vi "CountShantenWithoutEye.vi"(1 "HandCount":u16[](array[numeric])) -> (0 "shanten":u16)   [LabVIEW 2025]
panel:
  in  "VI Refnum":refnum<vi>
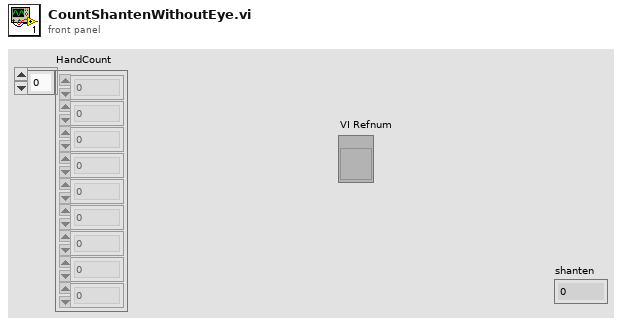
[diagram p1: front panel]
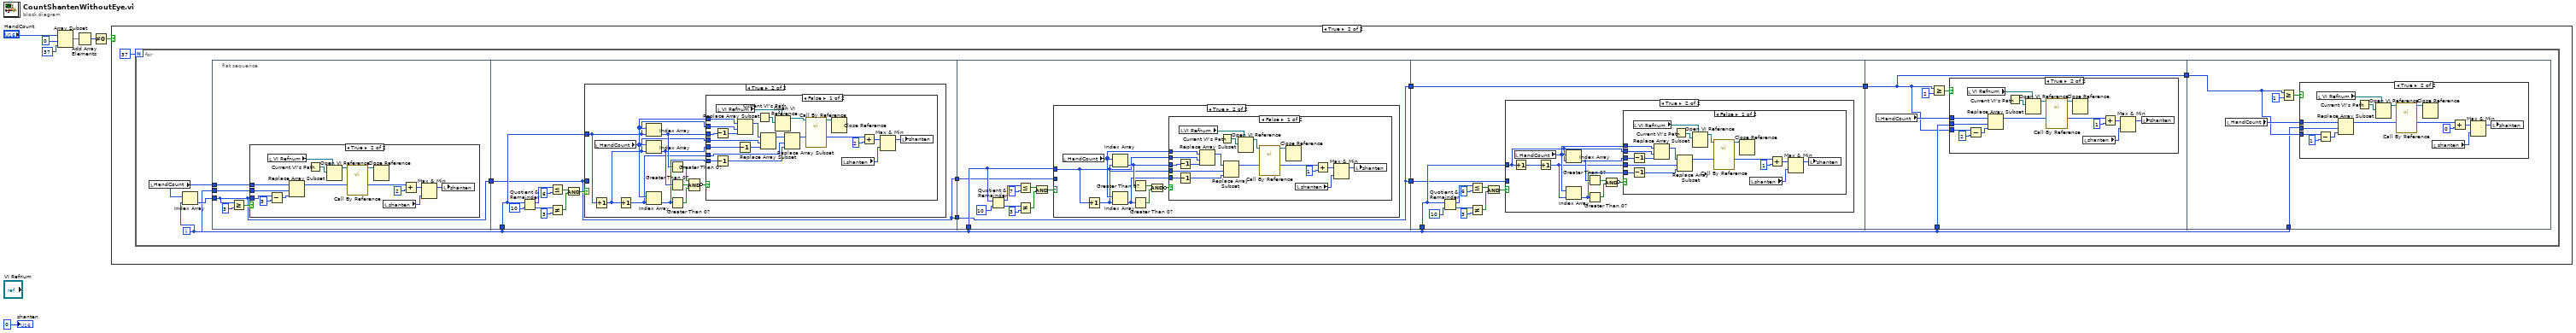
[diagram p0: block diagram]
diagram:
  n1 = Array Subset(array="HandCount", index=0, length=37) -> (w4:u16[])
  n2 = Add Array Elements(numeric array=w4) -> (sum=w2:u16)
  n3 = Not Equal To 0?(x=w2) -> (x != 0?=w3:bool)
  n4 = case shown="True" w3 {
    frame False {
    }
    frame True {
      n5 = for {
        N: 37 -> [_]
        i -> [w9]
        n6 = local read "HandCount"() -> (w16:u16[])
        n7 = Index Array(array=w16, index=w9) -> (element=w18:u16)
        n8 = flat-sequence {
          tunnel: w18 -> [w19]
          tunnel: [w19] -> w17
          tunnel: w16 -> [w21]
          tunnel: w9 -> [w20]
          tunnel: w17 -> [w39]
          tunnel: w9 -> [w41]
          tunnel: [w39] -> w15
          tunnel: [w39] -> w13
          tunnel: w9 -> [w84]
          tunnel: w15 -> [w83]
          tunnel: [w82] -> w14
          tunnel: w13 -> [w82]
          tunnel: [w82] -> w11
          tunnel: w9 -> [w121]
          tunnel: w14 -> [w120]
          tunnel: [w119] -> w12
          tunnel: w11 -> [w119]
          tunnel: w12 -> [w157]
          tunnel: w9 -> [w158]
          tunnel: [w157] -> w10
          tunnel: w10 -> [w178]
          tunnel: w9 -> [w177]
          frame #0 {
            n9 = Greater Or Equal?(x=w19, y=3) -> (x >= y?=w23:bool)
            n10 = case shown="True" w23 {
              tunnel: w21 -> [_ w38]
              tunnel: w20 -> [_ w37]
              tunnel: w19 -> [_ w34]
              frame False {
              }
              frame True {
                n11 = local read "VI Refnum"() -> (w32:refnum<vi>)
                n12 = Subtract(x=w34, y=3) -> (x-y=w35:i32)
                n13 = Replace Array Subset(array=w38, new element=w35, index=w37) -> (w30:u16[])
                n14 = Current VI's Path() -> (path=w33:path)
                n15 = Open VI Reference(type specifier VI Refnum (for type only)=w32, vi path=w33) -> (vi reference=w31:refnum<vi>)  [unwired: 4 in, 1 out]
                n16 = call-by-ref "?"(reference=w31, "HandCount"=w30) -> (reference out=w29:refnum<vi>, "Numeric"=w27:u16)  [unwired: 1 in, 1 out]
                n17 = Close Reference(reference=w29) -> ()  [unwired: 1 in, 1 out]
                n18 = local read "shanten"() -> (w28:u16)
                n19 = Add(x=w27, y=2) -> (x+y=w25:i32)
                n20 = Max & Min(x=w25, y=w28) -> (max(x,y)=w24:i32)  [unwired: 1 out]
                n21 = local write "shanten"(w24) -> ()
              }
            }
          }
          frame #1 {
            n22 = Quotient & Remainder(x=w41, y=10) -> (x-y*floor(x/y)=w47:i32, floor(x/y)=w45:i32)
            n23 = Less Or Equal?(x=w47, y=6) -> (x <= y?=w43:bool)
            n24 = Not Equal?(x=w45, y=3) -> (x != y?=w42:bool)
            n25 = And(x=w43, y=w42) -> (x .and. y?=w40:bool)
            n26 = case shown="True" w40 {
              tunnel: w39 -> [_ _]
              tunnel: w41 -> [_ w49]
              frame False {
              }
              frame True {
                n27 = Increment(x=w49) -> (x+1=w53:i32)
                n28 = local read "HandCount"() -> (w56:u16[])
                n29 = Increment(x=w53) -> (x+1=w51:i32)
                n30 = Index Array(array=w56, index=w49) -> (element=w55:u16)
                n31 = Index Array(array=w56, index=w53) -> (element=w54:u16)
                n32 = Index Array(array=w56, index=w51) -> (element=w52:u16)
                n33 = Greater Than 0?(x=w55) -> (x > 0?=w59:bool)
                n34 = Greater Than 0?(x=w54) -> (x > 0?=w58:bool)
                n35 = Greater Than 0?(x=w52) -> (x > 0?=w57:bool)
                n36 = Compound Arithmetic op=AND(w59, w58, w57) -> (invert w50:bool)
                n37 = case shown="False" w50 {
                  tunnel: w56 -> [w79 _]
                  tunnel: w55 -> [w75 _]
                  tunnel: w54 -> [w74 _]
                  tunnel: w53 -> [w73 _]
                  tunnel: w52 -> [w72 _]
                  tunnel: w51 -> [w71 _]
                  tunnel: w49 -> [w65 _]
                  frame False {
                    n38 = Decrement(x=w75) -> (x-1=w78:u16)
                    n39 = Decrement(x=w72) -> (x-1=w76:u16)
                    n40 = local read "VI Refnum"() -> (w70:refnum<vi>)
                    n41 = Replace Array Subset(array=w79, new element=w78, index=w65) -> (w81:u16[])
                    n42 = Decrement(x=w74) -> (x-1=w77:u16)
                    n43 = Current VI's Path() -> (path=w67:path)
                    n44 = Replace Array Subset(array=w81, new element=w77, index=w73) -> (w80:u16[])
                    n45 = Open VI Reference(type specifier VI Refnum (for type only)=w70, vi path=w67) -> (vi reference=w69:refnum<vi>)  [unwired: 4 in, 1 out]
                    n46 = Replace Array Subset(array=w80, new element=w76, index=w71) -> (w66:u16[])
                    n47 = call-by-ref "?"(reference=w69, "HandCount"=w66) -> (reference out=w68:refnum<vi>, "Numeric"=w60:u16)  [unwired: 1 in, 1 out]
                    n48 = Close Reference(reference=w68) -> ()  [unwired: 1 in, 1 out]
                    n49 = local read "shanten"() -> (w64:u16)
                    n50 = Add(x=w60, y=2) -> (x+y=w63:i32)
                    n51 = Max & Min(x=w63, y=w64) -> (max(x,y)=w62:i32)  [unwired: 1 out]
                    n52 = local write "shanten"(w62) -> ()
                  }
                  frame True {
                  }
                }
              }
            }
          }
          frame #2 {
            n53 = Quotient & Remainder(x=w84, y=10) -> (x-y*floor(x/y)=w86:i32, floor(x/y)=w88:i32)
            n54 = Less Or Equal?(x=w86, y=7) -> (x <= y?=w90:bool)
            n55 = Not Equal?(x=w88, y=3) -> (x != y?=w91:bool)
            n56 = And(x=w90, y=w91) -> (x .and. y?=w92:bool)
            n57 = case shown="True" w92 {
              tunnel: w83 -> [_ _]
              tunnel: w84 -> [_ w93]
              frame False {
              }
              frame True {
                n58 = local read "HandCount"() -> (w98:u16[])
                n59 = Increment(x=w93) -> (x+1=w95:i32)
                n60 = Index Array(array=w98, index=w93) -> (element=w97:u16)
                n61 = Index Array(array=w98, index=w95) -> (element=w96:u16)
                n62 = Greater Than 0?(x=w97) -> (x > 0?=w100:bool)
                n63 = Greater Than 0?(x=w96) -> (x > 0?=w99:bool)
                n64 = Compound Arithmetic op=AND(w100, w99) -> (invert w94:bool)
                n65 = case shown="False" w94 {
                  tunnel: w98 -> [w117 _]
                  tunnel: w97 -> [w114 _]
                  tunnel: w96 -> [w113 _]
                  tunnel: w95 -> [w112 _]
                  tunnel: w93 -> [w107 _]
                  frame False {
                    n66 = Decrement(x=w114) -> (x-1=w116:u16)
                    n67 = Decrement(x=w113) -> (x-1=w115:u16)
                    n68 = local read "VI Refnum"() -> (w111:refnum<vi>)
                    n69 = Replace Array Subset(array=w117, new element=w116, index=w107) -> (w118:u16[])
                    n70 = Current VI's Path() -> (path=w108:path)
                    n71 = Replace Array Subset(array=w118, new element=w115, index=w112) -> (w101:u16[])
                    n72 = Open VI Reference(type specifier VI Refnum (for type only)=w111, vi path=w108) -> (vi reference=w110:refnum<vi>)  [unwired: 4 in, 1 out]
                    n73 = call-by-ref "?"(reference=w110, "HandCount"=w101) -> (reference out=w109:refnum<vi>, "Numeric"=w102:u16)  [unwired: 1 in, 1 out]
                    n74 = Close Reference(reference=w109) -> ()  [unwired: 1 in, 1 out]
                    n75 = local read "shanten"() -> (w106:u16)
                    n76 = Add(x=w102, y=1) -> (x+y=w105:i32)
                    n77 = Max & Min(x=w105, y=w106) -> (max(x,y)=w104:i32)  [unwired: 1 out]
                    n78 = local write "shanten"(w104) -> ()
                  }
                  frame True {
                  }
                }
              }
            }
          }
          frame #3 {
            n79 = Quotient & Remainder(x=w121, y=10) -> (x-y*floor(x/y)=w128:i32, floor(x/y)=w126:i32)
            n80 = Less Or Equal?(x=w128, y=6) -> (x <= y?=w124:bool)
            n81 = Not Equal?(x=w126, y=3) -> (x != y?=w123:bool)
            n82 = And(x=w124, y=w123) -> (x .and. y?=w122:bool)
            n83 = case shown="True" w122 {
              tunnel: w120 -> [_ _]
              tunnel: w121 -> [_ w132]
              frame False {
              }
              frame True {
                n84 = Increment(x=w132) -> (x+1=w131:i32)
                n85 = local read "HandCount"() -> (w136:u16[])
                n86 = Increment(x=w131) -> (x+1=w130:i32)
                n87 = Index Array(array=w136, index=w132) -> (element=w135:u16)
                n88 = Index Array(array=w136, index=w130) -> (element=w134:u16)
                n89 = Greater Than 0?(x=w135) -> (x > 0?=w138:bool)
                n90 = Greater Than 0?(x=w134) -> (x > 0?=w137:bool)
                n91 = Compound Arithmetic op=AND(w138, w137) -> (invert w133:bool)
                n92 = case shown="False" w133 {
                  tunnel: w136 -> [w155 _]
                  tunnel: w135 -> [w152 _]
                  tunnel: w134 -> [w151 _]
                  tunnel: w130 -> [w150 _]
                  tunnel: w132 -> [w145 _]
                  frame False {
                    n93 = Decrement(x=w152) -> (x-1=w154:u16)
                    n94 = Decrement(x=w151) -> (x-1=w153:u16)
                    n95 = local read "VI Refnum"() -> (w149:refnum<vi>)
                    n96 = Replace Array Subset(array=w155, new element=w154, index=w145) -> (w156:u16[])
                    n97 = Current VI's Path() -> (path=w146:path)
                    n98 = Replace Array Subset(array=w156, new element=w153, index=w150) -> (w139:u16[])
                    n99 = Open VI Reference(type specifier VI Refnum (for type only)=w149, vi path=w146) -> (vi reference=w148:refnum<vi>)  [unwired: 4 in, 1 out]
                    n100 = call-by-ref "?"(reference=w148, "HandCount"=w139) -> (reference out=w147:refnum<vi>, "Numeric"=w140:u16)  [unwired: 1 in, 1 out]
                    n101 = Close Reference(reference=w147) -> ()  [unwired: 1 in, 1 out]
                    n102 = local read "shanten"() -> (w144:u16)
                    n103 = Add(x=w140, y=1) -> (x+y=w143:i32)
                    n104 = Max & Min(x=w143, y=w144) -> (max(x,y)=w142:i32)  [unwired: 1 out]
                    n105 = local write "shanten"(w142) -> ()
                  }
                  frame True {
                  }
                }
              }
            }
          }
          frame #4 {
            n106 = local read "HandCount"() -> (w159:u16[])
            n107 = Greater Or Equal?(x=w157, y=2) -> (x >= y?=w161:bool)
            n108 = case shown="True" w161 {
              tunnel: w159 -> [_ w176]
              tunnel: w158 -> [_ w175]
              tunnel: w157 -> [_ w172]
              frame False {
              }
              frame True {
                n109 = local read "VI Refnum"() -> (w170:refnum<vi>)
                n110 = Subtract(x=w172, y=2) -> (x-y=w173:i32)
                n111 = Replace Array Subset(array=w176, new element=w173, index=w175) -> (w168:u16[])
                n112 = Current VI's Path() -> (path=w171:path)
                n113 = Open VI Reference(type specifier VI Refnum (for type only)=w170, vi path=w171) -> (vi reference=w169:refnum<vi>)  [unwired: 4 in, 1 out]
                n114 = call-by-ref "?"(reference=w169, "HandCount"=w168) -> (reference out=w167:refnum<vi>, "Numeric"=w165:u16)  [unwired: 1 in, 1 out]
                n115 = Close Reference(reference=w167) -> ()  [unwired: 1 in, 1 out]
                n116 = local read "shanten"() -> (w166:u16)
                n117 = Add(x=w165, y=1) -> (x+y=w163:i32)
                n118 = Max & Min(x=w163, y=w166) -> (max(x,y)=w162:i32)  [unwired: 1 out]
                n119 = local write "shanten"(w162) -> ()
              }
            }
          }
          frame #5 {
            n120 = local read "HandCount"() -> (w181:u16[])
            n121 = Greater Or Equal?(x=w178, y=1) -> (x >= y?=w179:bool)
            n122 = case shown="True" w179 {
              tunnel: w181 -> [_ w196]
              tunnel: w177 -> [_ w195]
              tunnel: w178 -> [_ w192]
              frame False {
              }
              frame True {
                n123 = local read "VI Refnum"() -> (w190:refnum<vi>)
                n124 = Subtract(x=w192, y=1) -> (x-y=w193:i32)
                n125 = Replace Array Subset(array=w196, new element=w193, index=w195) -> (w188:u16[])
                n126 = Current VI's Path() -> (path=w191:path)
                n127 = Open VI Reference(type specifier VI Refnum (for type only)=w190, vi path=w191) -> (vi reference=w189:refnum<vi>)  [unwired: 4 in, 1 out]
                n128 = call-by-ref "?"(reference=w189, "HandCount"=w188) -> (reference out=w187:refnum<vi>, "Numeric"=w185:u16)  [unwired: 1 in, 1 out]
                n129 = Close Reference(reference=w187) -> ()  [unwired: 1 in, 1 out]
                n130 = local read "shanten"() -> (w186:u16)
                n131 = Add(x=w185, y=0) -> (x+y=w183:i32)
                n132 = Max & Min(x=w183, y=w186) -> (max(x,y)=w182:i32)  [unwired: 1 out]
                n133 = local write "shanten"(w182) -> ()
              }
            }
          }
        }
      }
    }
  }
  "shanten" <- u16 0 ("Numeric")
